vi "Write Publishers.vi"(8 "error in (no error)":errorcluster, 10 "Publishers":refnum<class "CIF_NIChn_Fifo_U8.lvclass">[](array[class]), 11 "CIF_Fifo_U8_Multi in":refnum<class "CIF_Fifo_U8_Multi.lvclass">) -> (0 "error out":errorcluster, 3 "CIF_Fifo_U8_Multi out":refnum<class "CIF_Fifo_U8_Multi.lvclass">)   [LabVIEW 2021, in "CIF_Fifo_U8_Multi.lvclass"]
uses:
  CIF_Fifo_U8_Multi.lvclass
  CIF_Fifo_U8_Multi.lvclass/CIF_Fifo_U8_Multi.ctl
  FIFO_U8/CIF_NIChn_Fifo_U8.lvclass
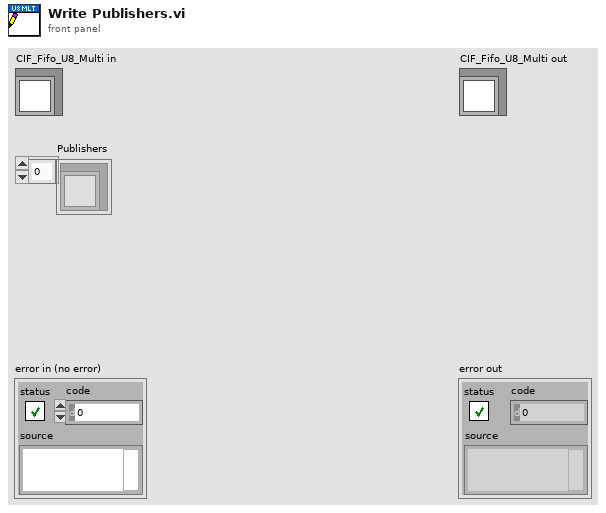
[diagram p1: front panel]
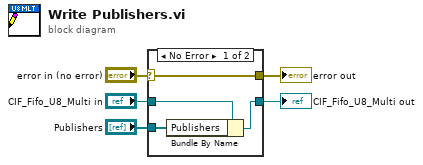
[diagram p0: block diagram]
diagram:
  n1 = case shown="No Error" "error in (no error)" {
    selector: "error in (no error)" -> [w9 w10]
    tunnel: [w9 w10] -> w4
    tunnel: [w7 w11] -> w2
    tunnel: "CIF_Fifo_U8_Multi in" -> [w8 w11]
    tunnel: "Publishers" -> [w6 _]
    frame No Error {
      n2 = Bundle By Name(cluster=w8, "Publishers"=w6) -> (w7:refnum<class "CIF_Fifo_U8_Multi.lvclass">)
    }
    frame Error {
    }
  }
  "error out" <- w4
  "CIF_Fifo_U8_Multi out" <- w2
